vi "1. First-Order Polynomial Test.vi"(8 "error in (no error)":errorcluster) -> (0 "error out":errorcluster)   [LabVIEW 2014]
uses:
  PolyA class/PolyA.lvclass
  <vilib>/LabVIEW Open Source Project/Configuration Manager/Manager/Decompose KVPs.vi
  <vilib>/LabVIEW Open Source Project/Configuration Manager/Manager/Write.vi
  <vilib>/JKI/JKI SMO/SMO/SMO.lvclass
  <vilib>/LabVIEW Open Source Project/Configuration Manager/Cache/ConfigManager.Cache.lvclass
  <vilib>/LabVIEW Open Source Project/Configuration Manager/Manager/ConfigManager.lvclass
  <vilib>/addons/_JKI Toolkits/Caraya/classes/Test/Test.lvclass
  <vilib>/addons/_JKI Toolkits/Caraya/classes/Assert/Assert.lvclass
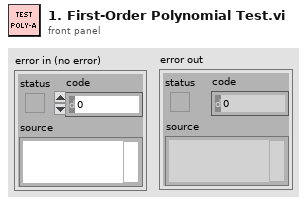
[diagram p1: front panel]
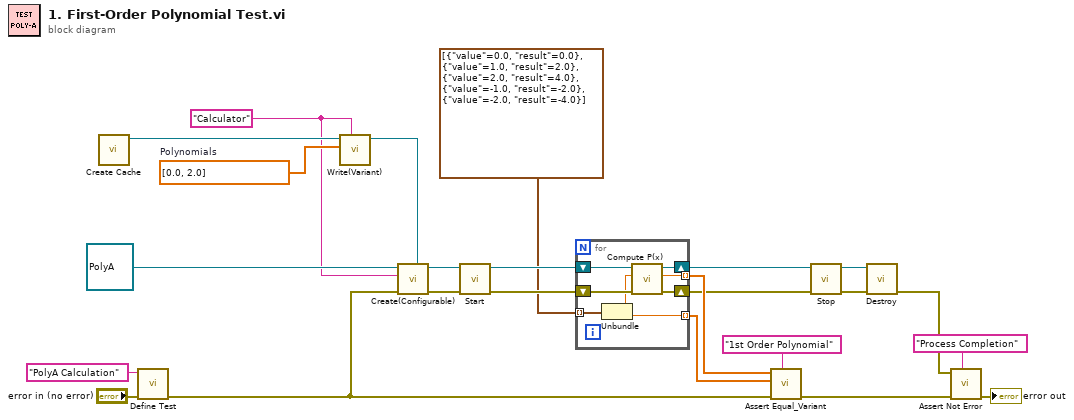
[diagram p0: block diagram]
diagram:
  w19 = dbl[] [0.0, 2.0]  # Polynomials
  w8 = "Calculator" ("Subsystem Name (optional)")
  n1 = call <vilib>:"Create Cache.vi"() -> ("ConfigManager.Cache"=w9:refnum<class "ConfigManager.Cache.lvclass">)  [unwired: 11 in]
  n2 = call <vilib>:"Define Test.vi"("error in (no error)"="error in (no error)", "Label (VI Title)"="PolyA Calculation") -> ("error out"=w16:errorcluster)  [unwired: 9 in]
  n3 = call <vilib>:"Write(Variant).vi"("Qualified Name"=w8, "value"=w19, "ConfigManager in"=w9) -> ("ConfigManager out"=w3:refnum<class "ConfigManager.Cache.lvclass">)  [unwired: 6 in, 2 out]
  n4 = call <vilib>:"Create(Configurable).vi"("ConfigManager"=w3, "error in (no error)"=w16, "Subsystem Name (optional)"=w8, "SMO"=refnum<class "PolyA.lvclass"> refnum ("PolyA.lvclass")) -> ("error out"=w23:errorcluster, "SMO out"=w24:refnum<class "PolyA.lvclass">)  [unwired: 5 in, 1 out]
  n5 = call <vilib>:"Start.vi"("error in (no error)"=w23, "SMO"=w24) -> ("error out"=w4:errorcluster, "SMO out"=w11:refnum<class "PolyA.lvclass">)  [unwired: 8 in]
  n6 = for {
    tunnel: [w31] -> w10 mode=indexing
    shift-right: [w30] -> w7
    shift-left: w11 -> [w32]
    shift-right: [w29] -> w6
    shift-left: w4 -> [w28]
    tunnel: cluster{"value":dbl, "result":dbl}[] [{"value"=0.0, "result"=0.0}, {"value"=1.0, "result"=2.0}, {"value"=2.0, "result"=4.0}, {"value"=-1.0, "result"=-2.0}, {"value"=-2.0, "result"=-4.0}] -> [w27] mode=indexing
    tunnel: [w25] -> w1 mode=indexing
    n7 = Unbundle(w27) -> ("value"=w26:dbl, "result"=w25:dbl)
    n8 = call "Compute P(x).vi"("error in (no error)"=w28, "x"=w26, "PolyA in"=w32) -> ("error out"=w29:errorcluster, "P(x)"=w31:dbl, "PolyA out"=w30:refnum<class "PolyA.lvclass">)  [unwired: 5 in, 1 out]
  }
  n9 = call <vilib>:"Assert Equal_Variant.vi"("Label"="1st Order Polynomial" ("Label (VI Title)"), "error in (no error)"=w16, "Y"=w1, "X"=w10) -> ("error out"=w5:errorcluster)  [unwired: 7 in]
  n10 = call <vilib>:"Stop.vi"("error in (no error)"=w6, "SMO"=w7) -> ("error out"=w21:errorcluster, "SMO out"=w22:refnum<class "PolyA.lvclass">)  [unwired: 8 in]
  n11 = call <vilib>:"Destroy.vi"("error in (no error)"=w21, "SMO"=w22) -> ("error out"=w15:errorcluster)  [unwired: 9 in]
  n12 = call <vilib>:"Assert Not Error.vi"("Label"="Process Completion" ("Label (VI Title)"), "error in (no error)"=w5, "Not Error?"=w15) -> ("error out"=→"error out":errorcluster)  [unwired: 8 in]
